vi "T7MOD_Read_FLOAT32_Registers.vi"(6 "Num Reg":i32=2, 8 "error in":errorcluster, 9 "Starting FLOAT32 Register":i32=55124, 10 "Remote Port":u16=502, 11 "Remote IP Address":string="192.168.1.15") -> (0 "error out":errorcluster, 1 "Read At":timestamp, 2 "Raw Data Read":u16[](array[numeric]), 3 "Read FLOAT32":sgl[](array[numeric]))   [LabVIEW 2016]
uses:
  Serial Link Layer/NI_Modbus_Cleaned/NI Modbus121Clean.llb/MB Ethernet Master Query Read Input Registers (poly).vi
panel:
  # "Output"
  # "TCP Parameters"
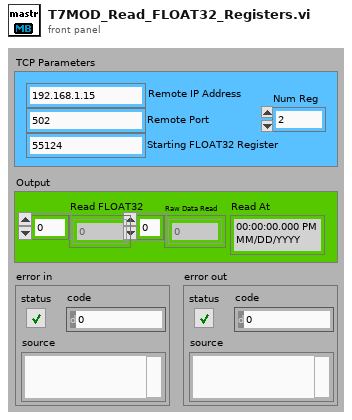
[diagram p1: front panel]
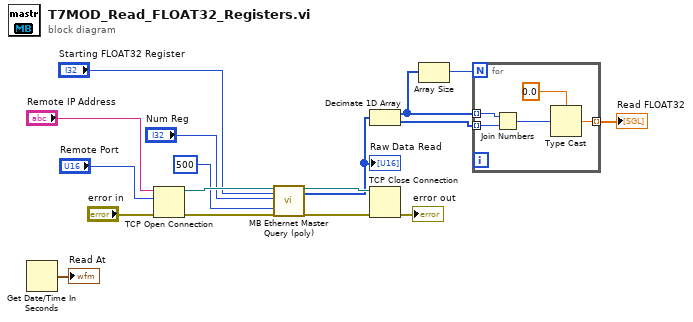
[diagram p0: block diagram]
diagram:
  n1 = Get Date/Time In Seconds() -> (seconds since 1Jan1904=→"Read At":timestamp)
  n2 = TCP Open Connection(address="Remote IP Address", remote port or service name="Remote Port", error in (no error)="error in") -> (connection ID=w15:refnum<k5>, error out=w14:errorcluster)  [unwired: 2 in]
  n3 = call-poly "MB Ethernet Master Query (poly).vi"("TCP Connection Refnum in"=w15, "Starting Address"="Starting FLOAT32 Register", "Quantity"="Num Reg", "Timeout"=500, "error in"=w14) -> ("TCP Connection Refnum (dup)"=w12:refnum<k5>, "Input Registers"=w6:u16[], "error out"=w13:errorcluster)  [unwired: 11 in, 1 out]
  "Raw Data Read" <- w6
  n4 = Decimate 1D Array(w6) -> (w2:u16[], w7:u16[])
  n5 = TCP Close Connection(connection ID=w12, error in (no error)=w13) -> (error out=→"error out":errorcluster)  [unwired: 2 out]
  n6 = Array Size(array=w2) -> (size(s)=w1:i32)
  n7 = for {
    N: w1 -> [_]
    tunnel: w2 -> [w22] mode=indexing
    tunnel: w7 -> [w21] mode=indexing
    tunnel: [w18] -> w5 mode=indexing
    n8 = Join Numbers(hi=w22, lo=w21) -> ((hi.lo)=w20:u32)
    n9 = Type Cast(type=sgl 0.0 ("type: FLOAT32"), x=w20) -> (*(type *) &x=w18:sgl)
  }
  "Read FLOAT32" <- w5
